vi "EJERCICIO 1.vi"() -> ()   [LabVIEW 2012]
panel:
  out "NUMERO INVERTIDO":dbl
  in  "INGRESE UN NUMERO":dbl
  # "INVERTIR NUMEROS"
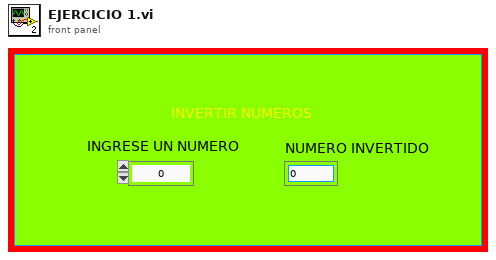
[diagram p1: front panel]
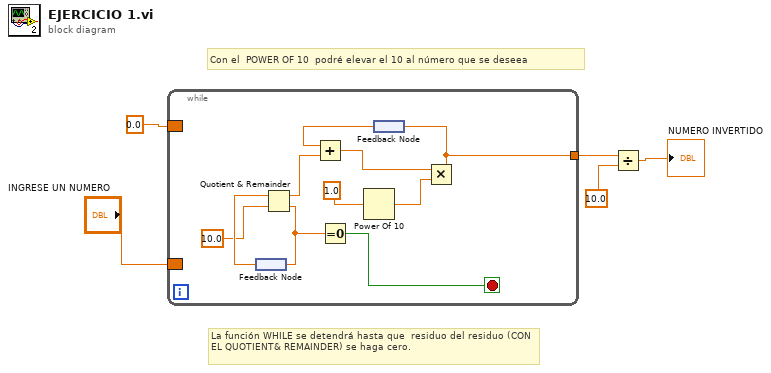
[diagram p0: block diagram]
diagram:
  # "Con el  POWER OF 10  podré elevar el 10 al número que se deseea"
  # "La función WHILE se detendrá hasta que  residuo del residuo (CON EL QUOTIENT& REMAINDER) se haga cero."
  n1 = while {
    tunnel: [w7] -> w3
    border: 0.0 -> [_]
    border: "INGRESE UN NUMERO" -> [_]
    stop <- w15 stop-if-true
    n2 = feedback #1() -> (w9:dbl)
    n3 = Quotient & Remainder(x=w9, y=10.0) -> (x-y*floor(x/y)=w13:dbl, floor(x/y)=w10:dbl)
    n4 = feedback-in #1(w10) -> ()
    n5 = Equal To 0?(x=w10) -> (x = 0?=w15:bool)
    n6 = Power Of 10(x=1.0) -> (10^x=w6:dbl)
    n7 = feedback #2() -> (w12:dbl)
    n8 = Add(x=w12, y=w13) -> (x+y=w11:dbl)
    n9 = Multiply(x=w11, y=w6) -> (x*y=w7:dbl)
    n10 = feedback-in #2(w7) -> ()
  }
  n11 = Divide(x=w3, y=10.0) -> (x/y=→"NUMERO INVERTIDO":dbl)
